vi "Get User Events.vi"   [LabVIEW 2011, in "Toolbar Control.lvclass"]
doc: "This is intended to be a merge VI on the palette\n\n-------------\nDeveloped by Brian Hoover (hooovahh)"
uses:
  Toolbar Control.lvclass
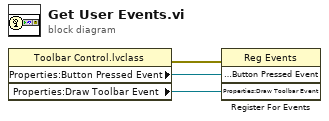
[diagram p0: block diagram]
diagram:
  n1 = property class="Toolbar Control.lvclass"() -> (error out=w3:errorcluster, "Properties:Button Pressed Event"=w2:refnum<user-event>, "Properties:Draw Toolbar Event"=w1:refnum<user-event>)  [unwired: 2 in, 1 out]
  n2 = register-events(error in=w3, w2, w1) -> ()  [unwired: 1 in, 2 out]
